vi "fgv_error.vi"(7 "cmd":T2, 11 "error 2":T1) -> (3 "error":T1)   [LabVIEW 2021]
uses:
  ctrl/ini-rw.ctl
  ctrl/error.ctl
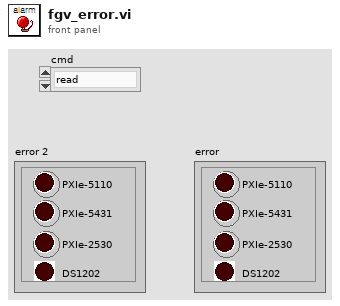
[diagram p1: front panel]
types:
  T1 = typedef "error.ctl" = cluster{"PXIe-5110":bool, "PXIe-5431":bool, "PXIe-2530":bool, "DS1202":bool}
  T2 = typedef "ini-rw.ctl" = enum16{"read", "write", "ini"}
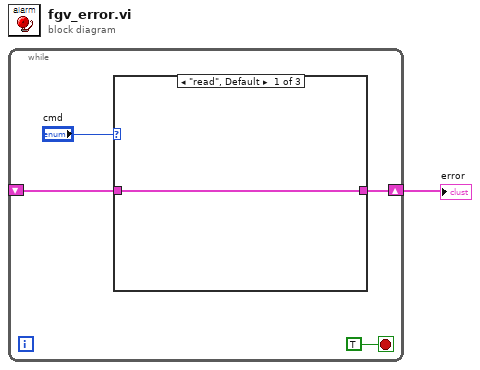
[diagram p0: block diagram]
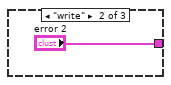
[diagram p2: hidden frame]
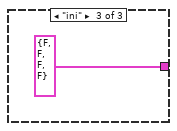
[diagram p3: hidden frame]
diagram:
  n1 = while {
    shift-right: [w3] -> w1
    shift-left: _ -> [w2]
    stop <- TRUE stop-if-true
    n2 = case shown="\"read\", Default" "cmd" {
      tunnel: [w6 "error 2" T1 {"PXIe-5110"=FALSE, "PXIe-5431"=FALSE, "PXIe-2530"=FALSE, "DS1202"=FALSE} ("error 2")] -> w3
      tunnel: w2 -> [w6 _ _]
      frame "read", Default {
      }
      frame "write" {
      }
      frame "ini" {
      }
    }
  }
  "error" <- w1
